vi "generate_cmd_string.vi"(4 "disk spinning":bool, 6 "disk position":bool, 7 "dichroic mirror":u16, 8 "error in (no error)":errorcluster, 9 "emission filter":u16, 10 "excitation filter":u16, 11 "port in":refnum<visa-resource-name>) -> (0 "error out":errorcluster, 2 "cmd string":string, 3 "port out":refnum<visa-resource-name>)   [LabVIEW 2016]
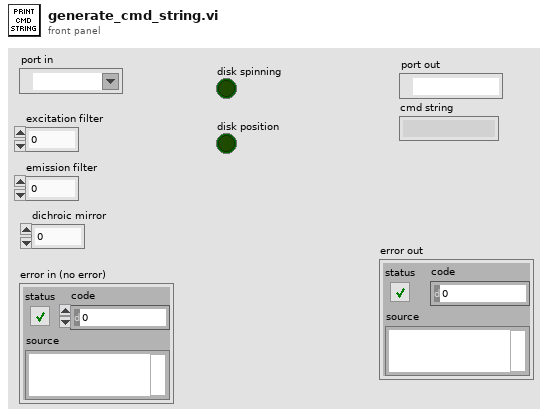
[diagram p1: front panel]
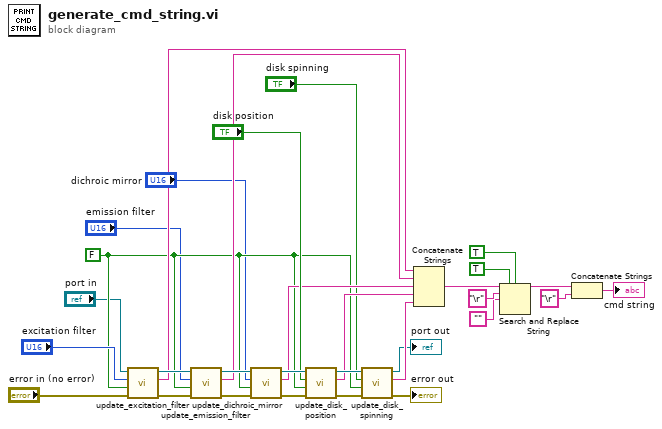
[diagram p0: block diagram]
diagram:
  w9 = FALSE ("commit?")
  n1 = call "update_excitation_filter.vi"("error in (no error)"="error in (no error)", "commit?"=w9, "excitation filter #"="excitation filter", "VISA resource name"="port in") -> ("error out"=w30:errorcluster, "cmd string"=w22:string, "VISA resource name out"=w31:refnum<visa-resource-name>)  [unwired: 1 out]
  n2 = call "update_emission_filter.vi"("error in (no error)"=w30, "commit?"=w9, "emission filter #"="emission filter", "VISA resource name"=w31) -> ("error out"=w29:errorcluster, "cmd string"=w21:string, "VISA resource name out"=w28:refnum<visa-resource-name>)  [unwired: 1 out]
  n3 = call "update_dichroic_mirror.vi"("error in (no error)"=w29, "commit?"=w9, "dichroic mirror #"="dichroic mirror", "VISA resource name"=w28) -> ("error out"=w26:errorcluster, "cmd string"=w20:string, "VISA resource name out"=w27:refnum<visa-resource-name>)  [unwired: 1 out]
  n4 = call "update_disk_position.vi"("error in (no error)"=w26, "commit?"=w9, "disk position"="disk position", "VISA resource name"=w27) -> ("error out"=w25:errorcluster, "cmd string"=w19:string, "VISA resource name out"=w24:refnum<visa-resource-name>)  [unwired: 1 out]
  n5 = call "update_disk_spinning.vi"("error in (no error)"=w25, "commit?"=w9, "disk spinning"="disk spinning", "VISA resource name"=w24) -> ("error out"=→"error out":errorcluster, "cmd string"=w18:string, "VISA resource name out"=→"port out":refnum<visa-resource-name>)  [unwired: 1 out]
  n6 = Concatenate Strings(w22, w21, w20, w19, w18) -> (w17:string)
  n7 = Search and Replace String(replace all?=TRUE ("replace all? (F)"), case sensitive?=TRUE ("ignore case? (F)"), input string=w17, search string="\r", replace string="") -> (result string=w12:string)  [unwired: 3 in, 3 out]
  n8 = Concatenate Strings(w12, "\r" ("string")) -> (→"cmd string":string)
